vi "Density controller (V).vi"() -> ()   [LabVIEW 2011]
uses:
  ADAM Client/Sub VIs/ADAM Controls/Address.ctl
  SubVI/Pumps_Valves_Dependencies_Global.vi
panel:
  in  "Density Calibration":bool
  in  "Fresh Fill Density (V)":dbl=3.734
  in  "Fresh Density (kg/m3)":dbl=1075.0
  in  "Brine Fill Density (V)":dbl=4.437
  in  "Brine Density (kg/m3)":dbl=1187.0
  out "Density Global Required (kg/m3)":dbl(graph)=1200.0
  in  "Read Density from Global":bool=TRUE
  in  "Sample Size Fresh Calibration":i32=20
  out "Fresh Reading Portable Density Meter":dbl=1075.0 format="%.2f"
  out "Fresh Reading Fill Density Meter":dbl=3.734
  out "Brine Reading Fill Density Meter":dbl=4.437
  out "Y intercept":dbl=480.109530583215
  out "Gradient":dbl=159.31721194879083
  out "Brine Reading Portable Density Meter":dbl=1187.0 format="%.2f"
  in  "Sample Size for Brine Calibration":i32=20
  out "Fill density meter reading (kg/m3)":dbl=1088.8605974395448
  in  "Backlash (Voltage required before Valve Moving)":dbl=0.3
  out "Density Measurement (kg/m3)":dbl(graph)=1088.8605974395448
  in  "K (Proportional Reposne for the system)":dbl=0.0005
  in  "Ki":dbl=0.5
  in  "Kd":dbl=0.0001
  out "Increment":dbl(graph)=0.13385721226173544
  out "Vout":dbl(graph)=8.0
  out "Demand":dbl(graph)=1.0
  out "Vout":dbl=8.0
  in  "Loop Delay":u32=5
  in  "Vmin (V)":dbl=4.0
  in  "Vmax (V)":dbl=8.0
  in  "Kp":dbl=0.0002
  in  "Density Required (kg/m3)":dbl=900.0
  in  "Measured Density (testing only)":dbl=1100.0
  in  "stop":bool
  # "For Density Calibration place tube into outlet and connect to Paar Density meter"
  # "If No Calibration Input Data Below"
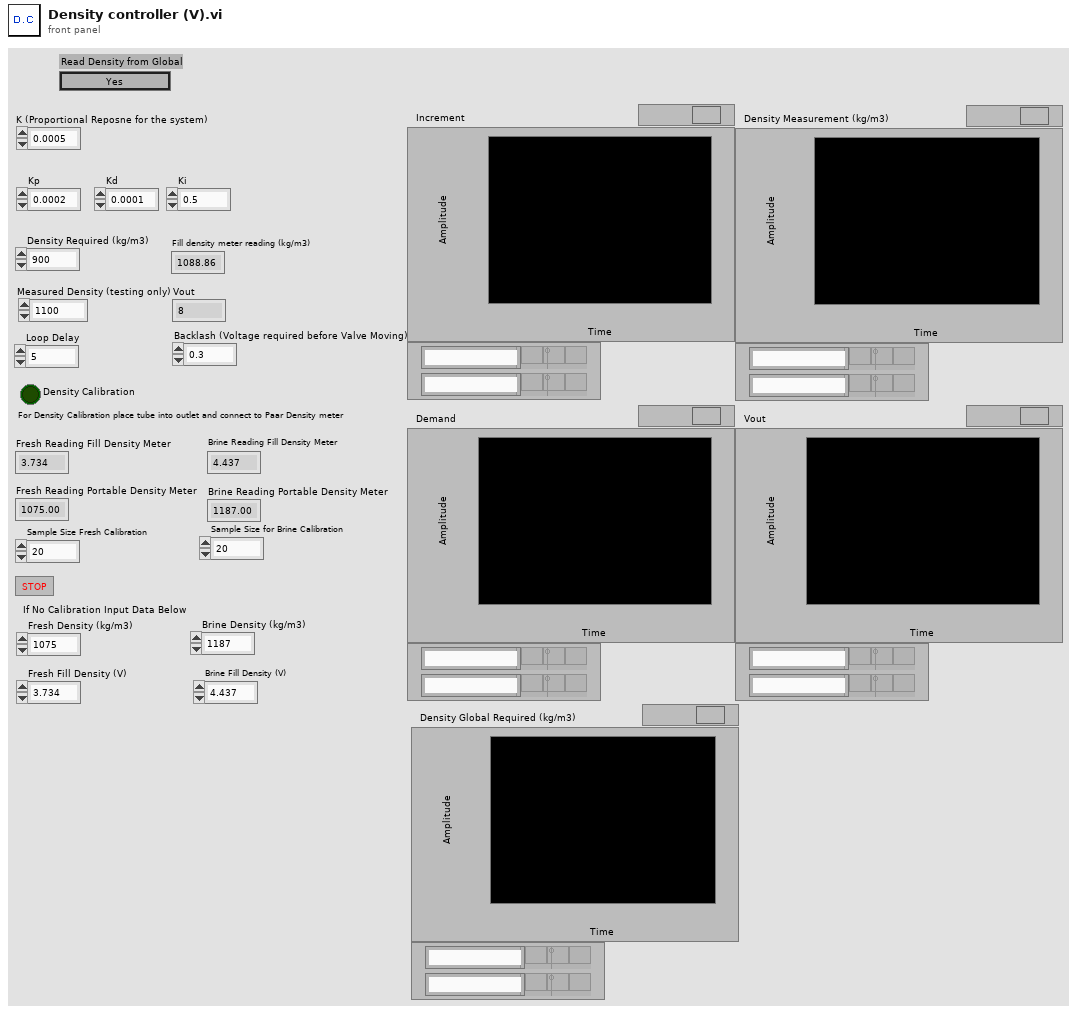
[diagram p1: front panel]
types:
  T1 = typedef "Address.ctl" = cluster{"Main":i32, "Ch.":i32, "Sub":i32, "Port Name":string}
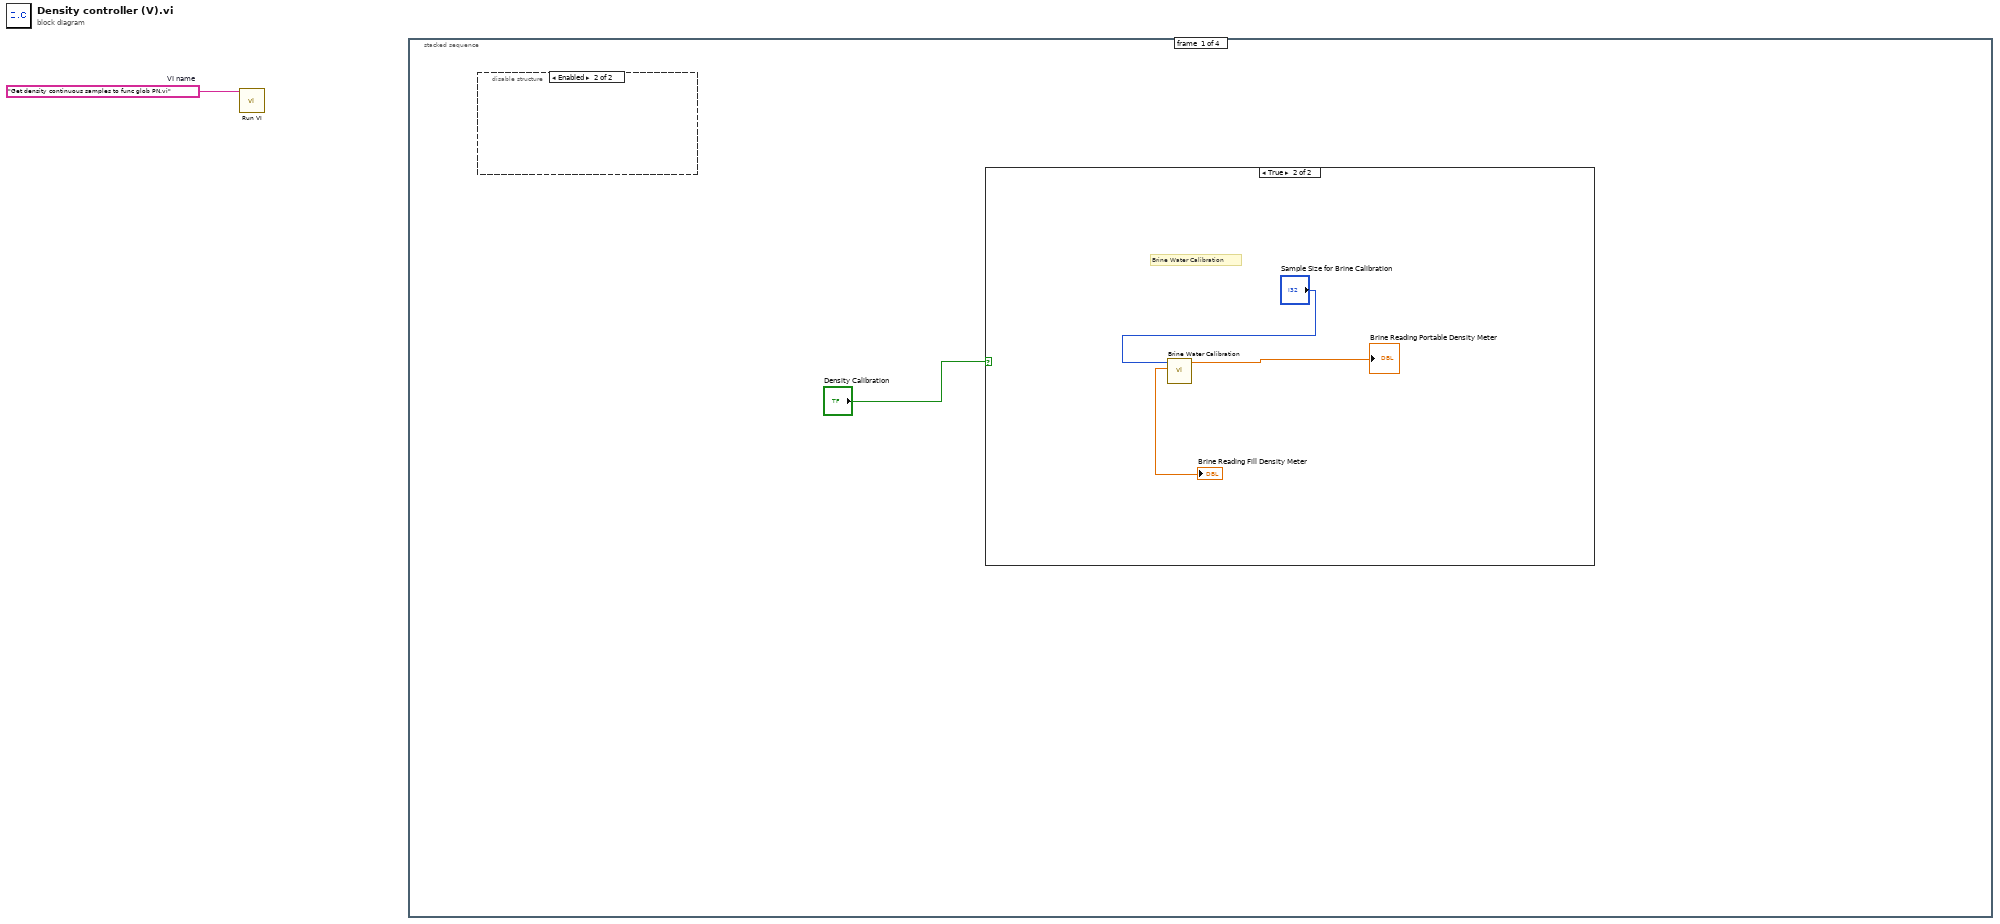
[diagram p0: block diagram]
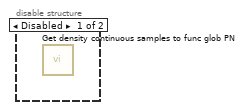
[diagram p2: hidden frame]
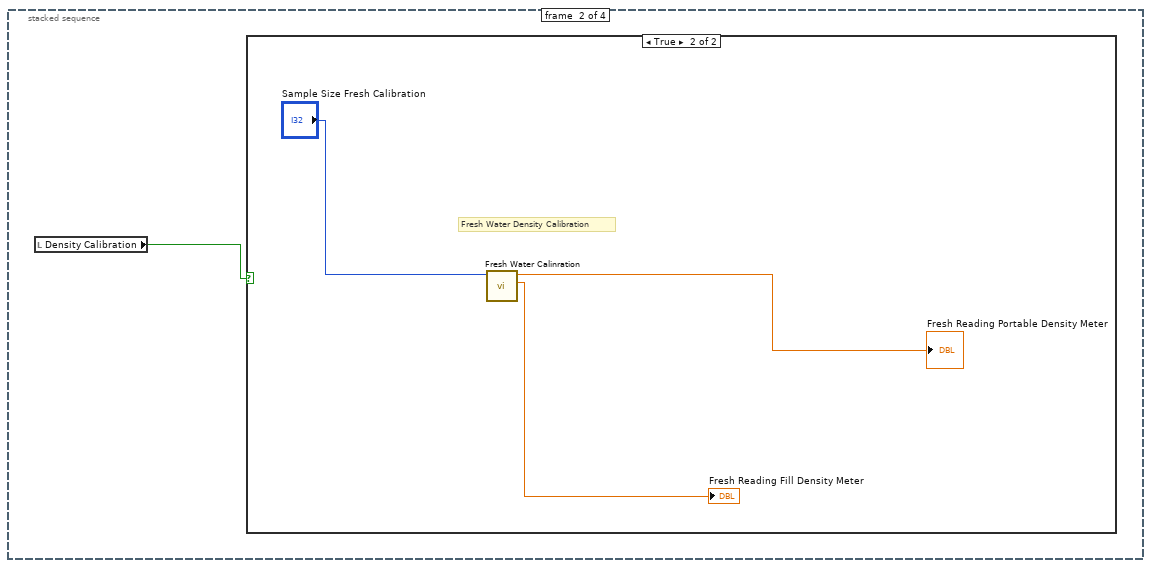
[diagram p4: hidden frame]
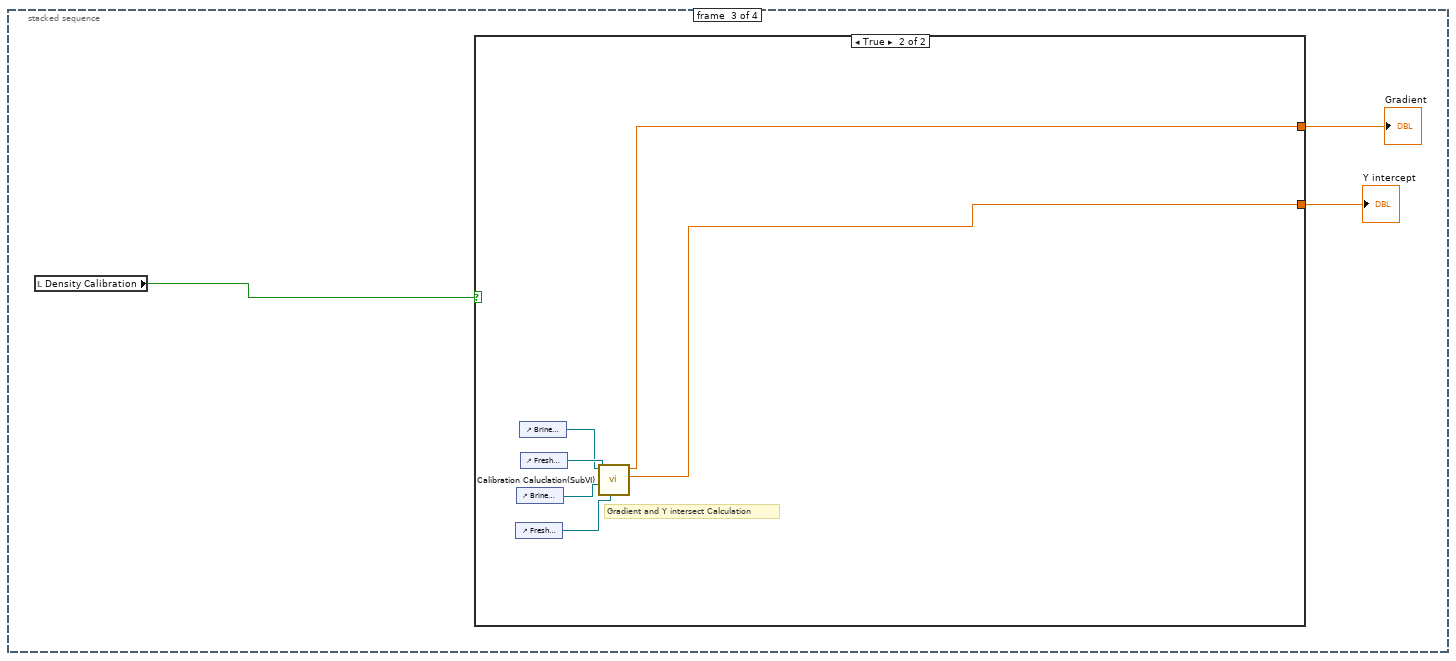
[diagram p6: hidden frame]
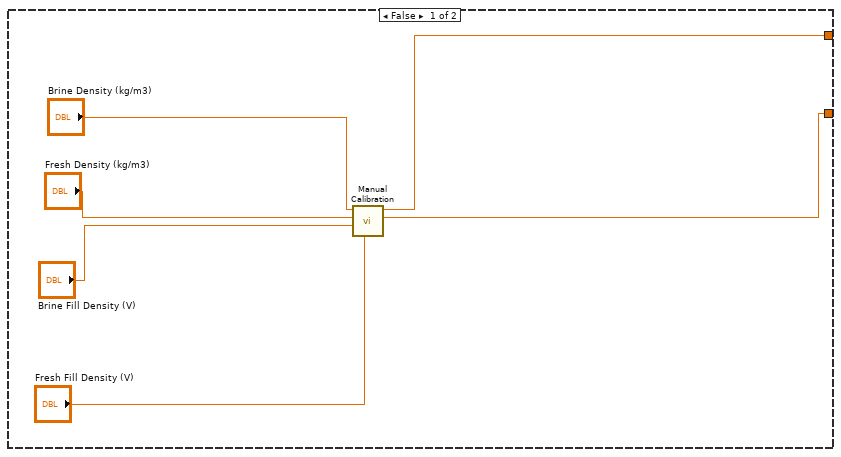
[diagram p7: hidden frame]
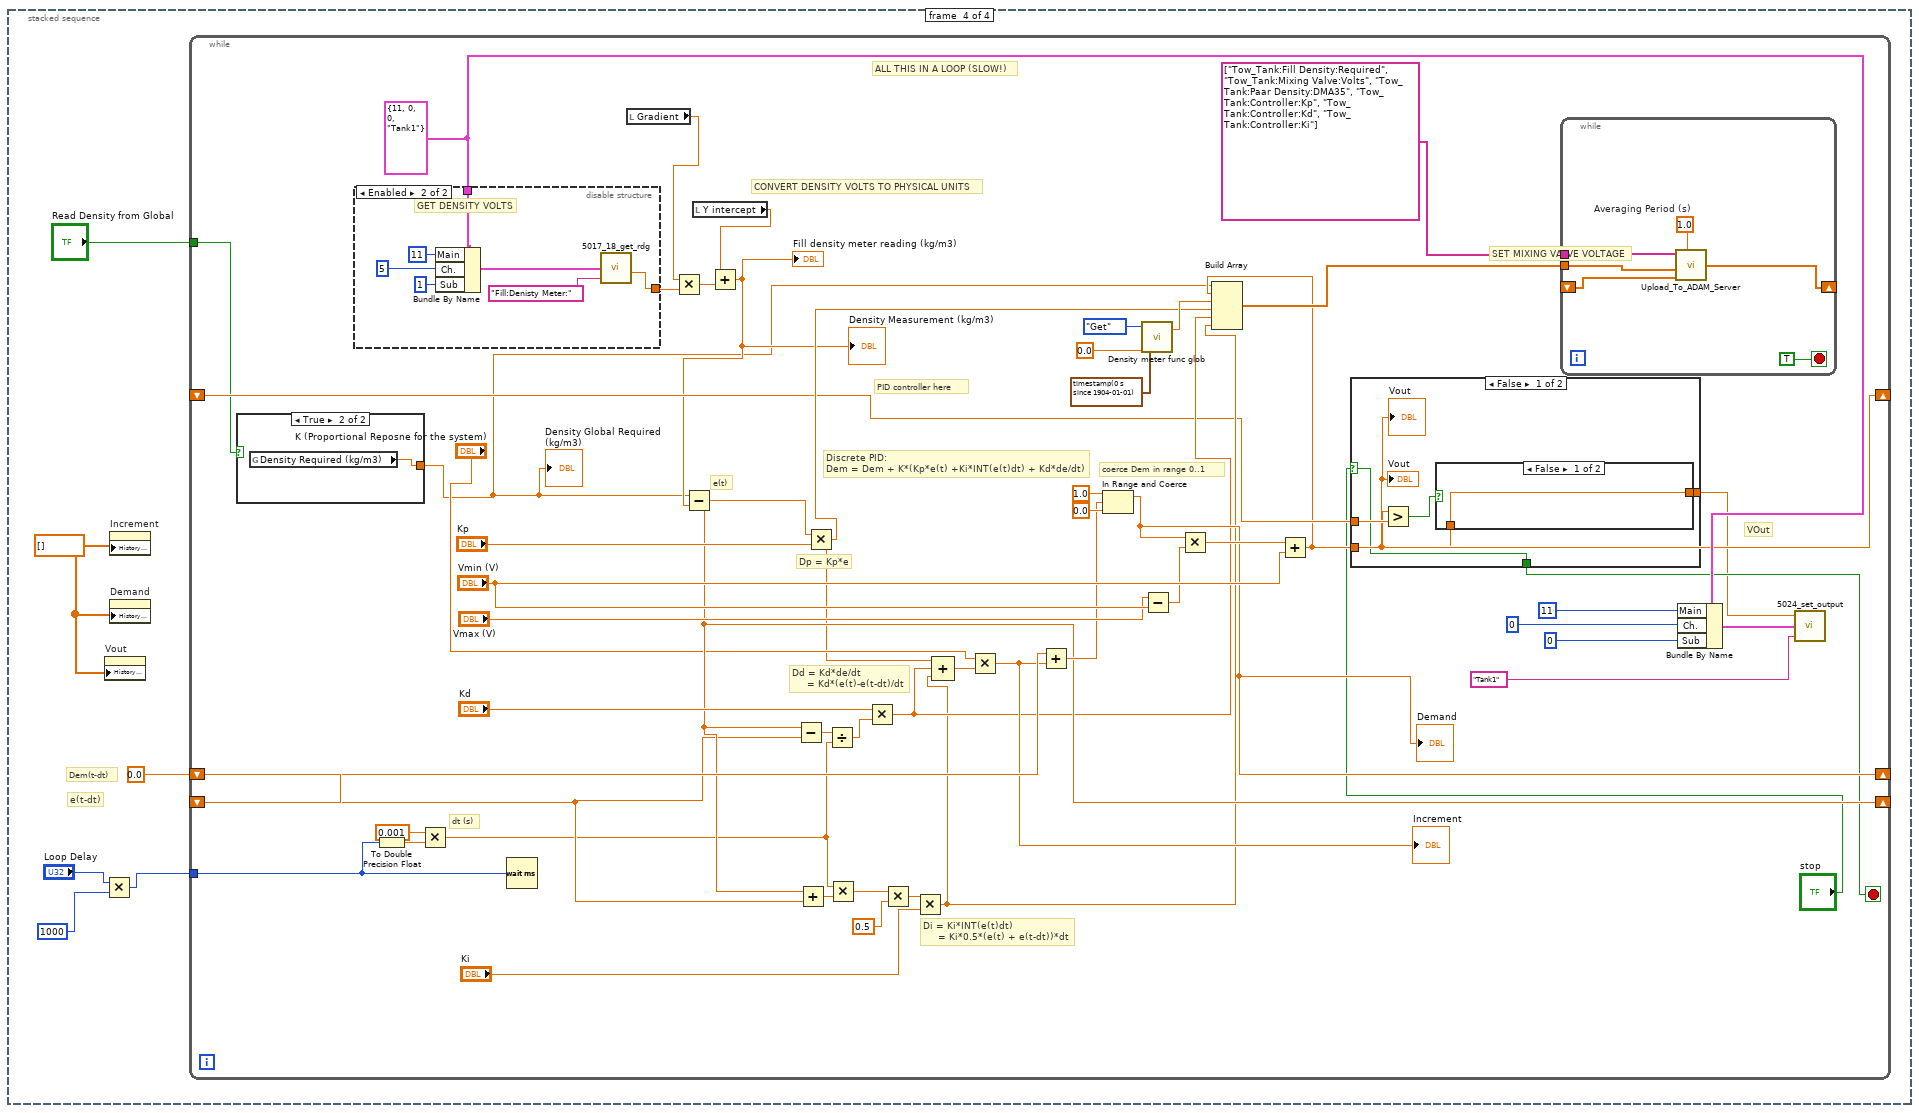
[diagram p8: hidden frame]
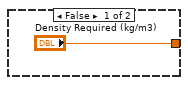
[diagram p9: hidden frame]
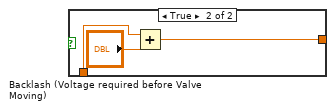
[diagram p10: hidden frame]
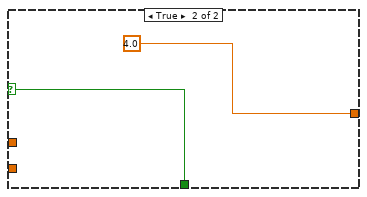
[diagram p11: hidden frame]
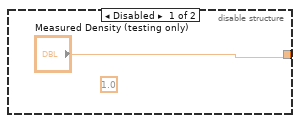
[diagram p12: hidden frame]
diagram:
  w1 = "Get density continuous samples to func glob PN.vi"  # VI name
  n1 = call "Run VI.vi"("VI name"=w1) -> ()  [unwired: 11 in]
  n2 = stacked-sequence {
    frame #0 {
      n3 = disable-structure shown="Enabled" {
        frame Disabled {
          n4 = call "Get density continuous samples to func glob PN.vi"() -> ()  [unwired: 3 in]
        }
        frame Enabled {
        }
      }
      n5 = case shown="True" "Density Calibration" {
        frame False {
        }
        frame True {
          # "Brine Water Calibration"
          n6 = call "Brine Water Calibration.vi"("Sample Size for Density Meter Reading"="Sample Size for Brine Calibration") -> ("Brine Reading Fill Density Meter"=→"Brine Reading Fill Density Meter":dbl, "Brine Reading Portable Density Meter"=→"Brine Reading Portable Density Meter":dbl)  [unwired: 9 in]
        }
      }
    }
    frame #1 {
      n7 = local read "Density Calibration"() -> (w6:bool)
      n8 = case shown="True" w6 {
        frame False {
        }
        frame True {
          # "Fresh Water Density Calibration"
          n9 = call "Fresh Water Calinration.vi"("Sample Size for Density Meter Reading  in"="Sample Size Fresh Calibration") -> ("Fresh Reading Fill Density Meter"=→"Fresh Reading Fill Density Meter":dbl, "Fresh Reading Portable Density Meter"=→"Fresh Reading Portable Density Meter":dbl)  [unwired: 9 in]
        }
      }
    }
    frame #2 {
      n10 = local read "Density Calibration"() -> (w12:bool)
      n11 = case shown="True" w12 {
        tunnel: [w13 w20] -> w11
        tunnel: [w14 w19] -> w10
        frame False {
          n12 = call "Manual Calibration.vi"("Fresh Fill Density (V)"="Fresh Fill Density (V)", "Brine Fill Density (V)"="Brine Fill Density (V)", "Fresh Density (kg/m3) 3"="Fresh Density (kg/m3)", "Brine Density (kg/m3)"="Brine Density (kg/m3)") -> ("Numeric 2"=w14:dbl, "Numeric"=w13:dbl)  [unwired: 6 in]
        }
        frame True {
          # "Gradient and Y intersect Calculation"
          n13 = control-ref of="Fresh Reading Portable Density Meter"() -> (w24:refnum<vi>)
          n14 = control-ref of="Brine Reading Fill Density Meter"() -> (w23:refnum<vi>)
          n15 = control-ref of="Brine Reading Portable Density Meter"() -> (w21:refnum<vi>)
          n16 = control-ref of="Fresh Reading Fill Density Meter"() -> (w22:refnum<vi>)
          n17 = call "Calibration Caluclation(SubVI).vi"("reference in"=w24, "reference 3"=w23, "reference 4"=w22, "Digital in"=w21) -> ("Y intercept"=w19:dbl, "Gradient"=w20:dbl)  [unwired: 6 in]
        }
      }
      "Gradient" <- w11
      "Y intercept" <- w10
    }
    frame #3 {
      w30 = dbl[] [] ("History Data")
      w29 = 0.0 ("Actual Density (kg/m3) 2")
      # "e(t-dt)"
      # "Dem(t-dt)"
      n18 = Multiply(x="Loop Delay", y=u32 1000 ("loop delay 2")) -> (x*y=w28:u32)
      n19 = property on="Vout" class="WFChart (strict)"("History Data"=w30) -> ()  [unwired: 2 in, 2 out]
      n20 = property on="Increment" class="WFChart (strict)"("History Data"=w30) -> ()  [unwired: 2 in, 2 out]
      n21 = property on="Demand" class="WFChart (strict)"("History Data"=w30) -> ()  [unwired: 2 in, 2 out]
      n22 = while {
        shift-right: [w71] -> _
        shift-left: w29 -> [w64]
        shift-right: [w62] -> _
        shift-left: w29 -> [w61]
        tunnel: w28 -> [w70]
        shift-right: [w41] -> _
        shift-left: _ -> [w42]
        tunnel: "Read Density from Global" -> [w32]
        stop <- w39 stop-if-true
        w82 = T1 {"Main"=11, "Ch."=0, "Sub"=0, "Port Name"="Tank1"} ("Address (all reqd.)")
        # "Di = Ki*INT(e(t)dt)\n     = Ki*0.5*(e(t) + e(t-dt))*dt"
        # "Dd = Kd*de/dt\n     = Kd*(e(t)-e(t-dt)/dt"
        # "dt (s)"
        # "coerce Dem in range 0..1"
        # "Discrete PID:\nDem = Dem + K*(Kp*e(t) +Ki*INT(e(t)dt) + Kd*de/dt)"
        # "Dp = Kp*e"
        # "e(t)"
        # "ALL THIS IN A LOOP (SLOW!)"
        # "CONVERT DENSITY VOLTS TO PHYSICAL UNITS"
        # "PID controller here"
        # "VOut"
        # "SET MIXING VALVE VOLTAGE"
        n23 = case shown="True" w32 {
          tunnel: ["Density Required (kg/m3)" w86] -> w31
          frame False {
          }
          frame True {
            n24 = global read "Pumps_Valves_Dependencies_Global.vi" "Density Required (kg/m3)"() -> (w86:dbl)
          }
        }
        "Density Global Required (kg/m3)" <- w31
        n25 = disable-structure shown="Enabled" {
          disable-tunnel: w82 -> [_ w106]
          disable-tunnel: ["Measured Density (testing only)" w105] -> w37
          frame Disabled {
            (unwired) 1.0 ("x")
          }
          frame Enabled {
            # "GET DENSITY VOLTS"
            n26 = Bundle By Name(cluster=w106, "Main"=11, "Ch."=5, "Sub"=1) -> (w108:T1)
            n27 = call "5017_18_get_rdg.vi"("Address (all reqd.)"=w108, "Channel Name"="Fill:Denisty Meter:") -> ("Reading"=w105:dbl)  [unwired: 3 in, 1 out]
          }
        }
        n28 = To Double Precision Float(number=w70) -> (double precision float=w69:dbl)
        n29 = Multiply(x=0.001, y=w69) -> (x*y=w59:dbl)
        n30 = Wait (ms)(milliseconds to wait=w70) -> ()  [unwired: 1 out]
        n31 = local read "Gradient"() -> (w34:dbl)
        n32 = Multiply(x=w34, y=w37) -> (x*y=w36:dbl)
        n33 = local read "Y intercept"() -> (w33:dbl)
        n34 = Add(x=w33, y=w36) -> (x+y=w35:dbl)
        "Density Measurement (kg/m3)" <- w35
        "Fill density meter reading (kg/m3)" <- w35
        n35 = Subtract(x=w31, y=w35) -> (x-y=w62:dbl)
        n36 = Subtract(x=w62, y=w61) -> (x-y=w67:dbl)
        n37 = Add(x=w62, y=w61) -> (x+y=w60:dbl)
        n38 = Multiply(x=w62, y="Kp") -> (x*y=w45:dbl)
        n39 = Divide(x=w67, y=w59) -> (x/y=w66:dbl)
        n40 = Multiply(x=w59, y=w60) -> (x*y=w57:dbl)
        n41 = Multiply(x="Kd", y=w66) -> (x*y=w44:dbl)
        n42 = Multiply(x=w57, y=0.5 ("x")) -> (x*y=w56:dbl)
        n43 = Multiply(x=w56, y="Ki") -> (x*y=w43:dbl)
        n44 = Compound Arithmetic op=ADD(w45, w44, w43) -> (w54:dbl)
        n45 = Multiply(x="K (Proportional Reposne for the system)", y=w54) -> (x*y=w52:dbl)
        "Increment" <- w52
        n46 = Add(x=w64, y=w52) -> (x+y=w63:dbl)
        n47 = In Range and Coerce(upper limit=1.0, x=w63, lower limit=0.0) -> (coerced(x)=w71:dbl)  [unwired: 1 out]
        "Demand" <- w71
        n48 = call "Density meter func glob.vi"("Sample DateTime in"=timestamp(0 s since 1904-01-01), "Density in"=0.0, "Action"=enum16{"Get", "Set"}."Get") -> ("Density out"=w48:dbl)  [unwired: 1 out]
        n49 = Subtract(x="Vmax (V)", y="Vmin (V)") -> (x-y=w75:dbl)
        n50 = Multiply(x=w71, y=w75) -> (x*y=w74:dbl)
        n51 = Add(x=w74, y="Vmin (V)") -> (x+y=w41:dbl)
        n52 = Build Array(w31, w41, w48, w45, w44, w43) -> (w50:dbl[])
        n53 = case shown="False" "stop" {
          selector: "stop" -> [w87 w97]
          tunnel: w42 -> [w91 _]
          tunnel: w41 -> [w89 _]
          tunnel: [w88 4.0 ("x")] -> w38
          tunnel: [w87 w97] -> w39
          frame False {
            n54 = Greater?(x=w89, y=w91) -> (0:w90:bool)
            n55 = case shown="False" w90 {
              tunnel: w89 -> [w92 w95]
              tunnel: [w92 w94] -> w88
              frame False {
              }
              frame True {
                n56 = Add(x=w95, y="Backlash (Voltage required before Valve Moving)") -> (x+y=w94:dbl)
              }
            }
            "Vout" <- w89
            "Vout" <- w89
          }
          frame True {
          }
        }
        n57 = while {
          shift-right: [w102] -> _
          shift-left: _ -> [w99]
          tunnel: w50 -> [w101]
          tunnel: string[] ["Tow_Tank:Fill Density:Required", "Tow_Tank:Mixing Valve:Volts", "Tow_Tank:Paar Density:DMA35", "Tow_Tank:Controller:Kp", "Tow_Tank:Controller:Kd", "Tow_Tank:Controller:Ki"] -> [w98]
          stop <- TRUE stop-if-true
          w103 = 1.0  # Averaging Period (s)
          n58 = call "Upload_To_ADAM_Server.vi"("Averaging Period (s)"=w103, "Shift In"=w99, "Channel Values"=w101, "Channel Names"=w98) -> ("Shift Out"=w102:dbl[])  [unwired: 2 in]
        }
        n59 = Bundle By Name(cluster=w82, "Main"=11, "Ch."=0, "Sub"=0) -> (w83:T1)
        n60 = call "5024_set_output.vi"("Set to:"=w38, "Address (all reqd.)"=w83, "Channel Name"="Tank1" ("Port Name")) -> ()  [unwired: 2 in, 2 out]
      }
    }
  }
